vi "Resample signal to Fs.vi"(7 "fine":bool, 9 "Fs (3.072G)":dbl format="%#_6p", 10 "Signal rate":dbl=500000000.0 format="%#_6p", 11 "Signal in":dbl[](array[numeric])) -> (3 "Signal out":dbl[](array[numeric]))   [LabVIEW 2019]
doc: "Resamples imput signal from its defined rate to Fs"
uses:
  <vilib>/Analysis/1siggen.llb/Ramp Pattern by Samples.vi
  <vilib>/measure/maresamp.llb/Resample Waveform (single shot).vi
  <vilib>/measure/NI_MAPro.lvlib
  <vilib>/Analysis/NI_AALBase.lvlib
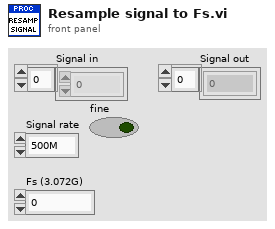
[diagram p1: front panel]
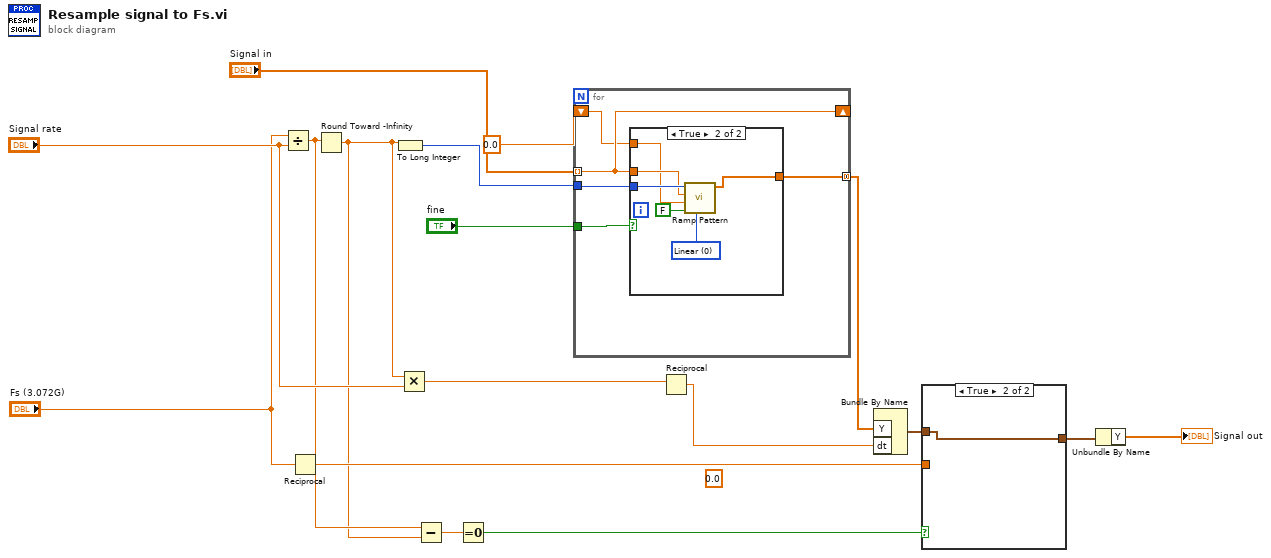
[diagram p0: block diagram]
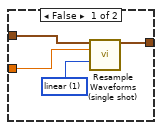
[diagram p2: hidden frame]
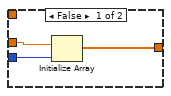
[diagram p3: hidden frame]
diagram:
  (unwired) 0.0 ("1/x")
  n1 = Divide(x="Fs (3.072G)", y="Signal rate") -> (x/y=w5:dbl)
  n2 = Reciprocal(x="Fs (3.072G)") -> (1/x=w11:dbl)
  n3 = Round Toward -Infinity(1:w5) -> (0:w4:dbl)
  n4 = To Long Integer(number=w4) -> (32bit integer=w12:i32)
  n5 = Multiply(x=w4, y="Signal rate") -> (x*y=w14:dbl)
  n6 = Subtract(x=w5, y=w4) -> (x-y=w3:dbl)
  n7 = Equal To 0?(x=w3) -> (x = 0?=w2:bool)
  n8 = for {
    tunnel: w12 -> [w22]
    tunnel: "Signal in" -> [w21] mode=indexing
    tunnel: [w19] -> w15 mode=concatenating
    shift-right: [w21] -> _
    shift-left: 0.0 ("floor(x): largest int <= x") -> [w20]
    tunnel: "fine" -> [w18]
    n9 = case shown="True" w18 {
      tunnel: w22 -> [w25 w31]
      tunnel: w21 -> [w24 w30]
      tunnel: w20 -> [_ w29]
      tunnel: [w23 w27] -> w19
      frame False {
        n10 = Initialize Array(w24, w25) -> (w23:dbl[])
      }
      frame True {
        w26 = u16 0 items=["Linear", "Logarithmic"] ("type")
        n11 = call-poly <vilib>:"Ramp Pattern.vi"("type"=w26, "exclude end?"=FALSE, "start"=w29, "end"=w30, "samples"=w31) -> ("Ramp Pattern"=w27:dbl[])  [unwired: 5 in, 1 out]
      }
    }
  }
  n12 = Reciprocal(x=w14) -> (1/x=w16:dbl)
  n13 = Bundle By Name("Y"=w15, "dt"=w16) -> (w7:waveform(dbl))  [unwired: 1 in]
  n14 = case shown="True" w2 {
    tunnel: w11 -> [w34 _]
    tunnel: [w33 w36] -> w8
    tunnel: w7 -> [w32 w36]
    frame False {
      w35 = u16 1 items=["coerce", "linear", "spline", "FIR filter"] ("interpolation mode")
      n15 = call-poly <vilib>:"Resample Waveforms (single shot).vi"("waveform in"=w32, "dt"=w34, "interpolation mode"=w35) -> ("resampled waveform out"=w33:waveform(dbl))  [unwired: 9 in, 3 out]
    }
    frame True {
    }
  }
  n16 = Unbundle By Name(w8) -> ("Y"=→"Signal out":dbl[])
